vi "PROYECTO_FINAL.vi"() -> ()   [LabVIEW 2026]
uses:
  <vilib>/Instr/_visa.llb/VISA Configure Serial Port (Instr).vi
panel:
  out "MONITOR SERIAL":string
  out "ASIENTO 2 Ocupado":bool
  out "ASIENTO 1 Ocupado":bool
  out "detenido":bool
  out "volcadura":bool
  out "Velocidad GPS":dbl
  out "Humedad":dbl
  out "Temp AHT":dbl
  out "Altitud":dbl
  out "Temp BMP":dbl
  out "Presión":dbl
  out "ROLL":dbl
  out "PITCH":dbl
  out "AZ":dbl
  out "AY":dbl
  out "AX":dbl
  in  "stop":bool
  # "PROYECTO FINAL"
  # "TÓPICOS AVANZADOS \nDE SENSORES"
  # "-GARCÍA PÉREZ VÍCTOR EDUARDO\n-FRAIRE MEZA ARIATNO TOMASSI\n-NAVA ÁVILA DAVID ISAAC"
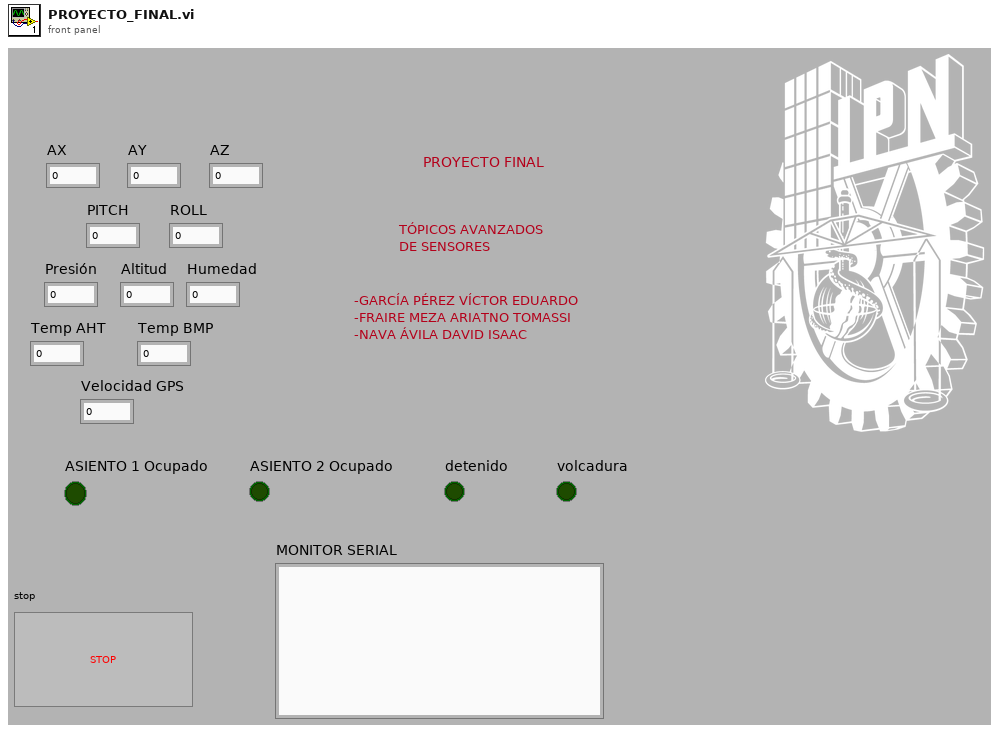
[diagram p1: front panel]
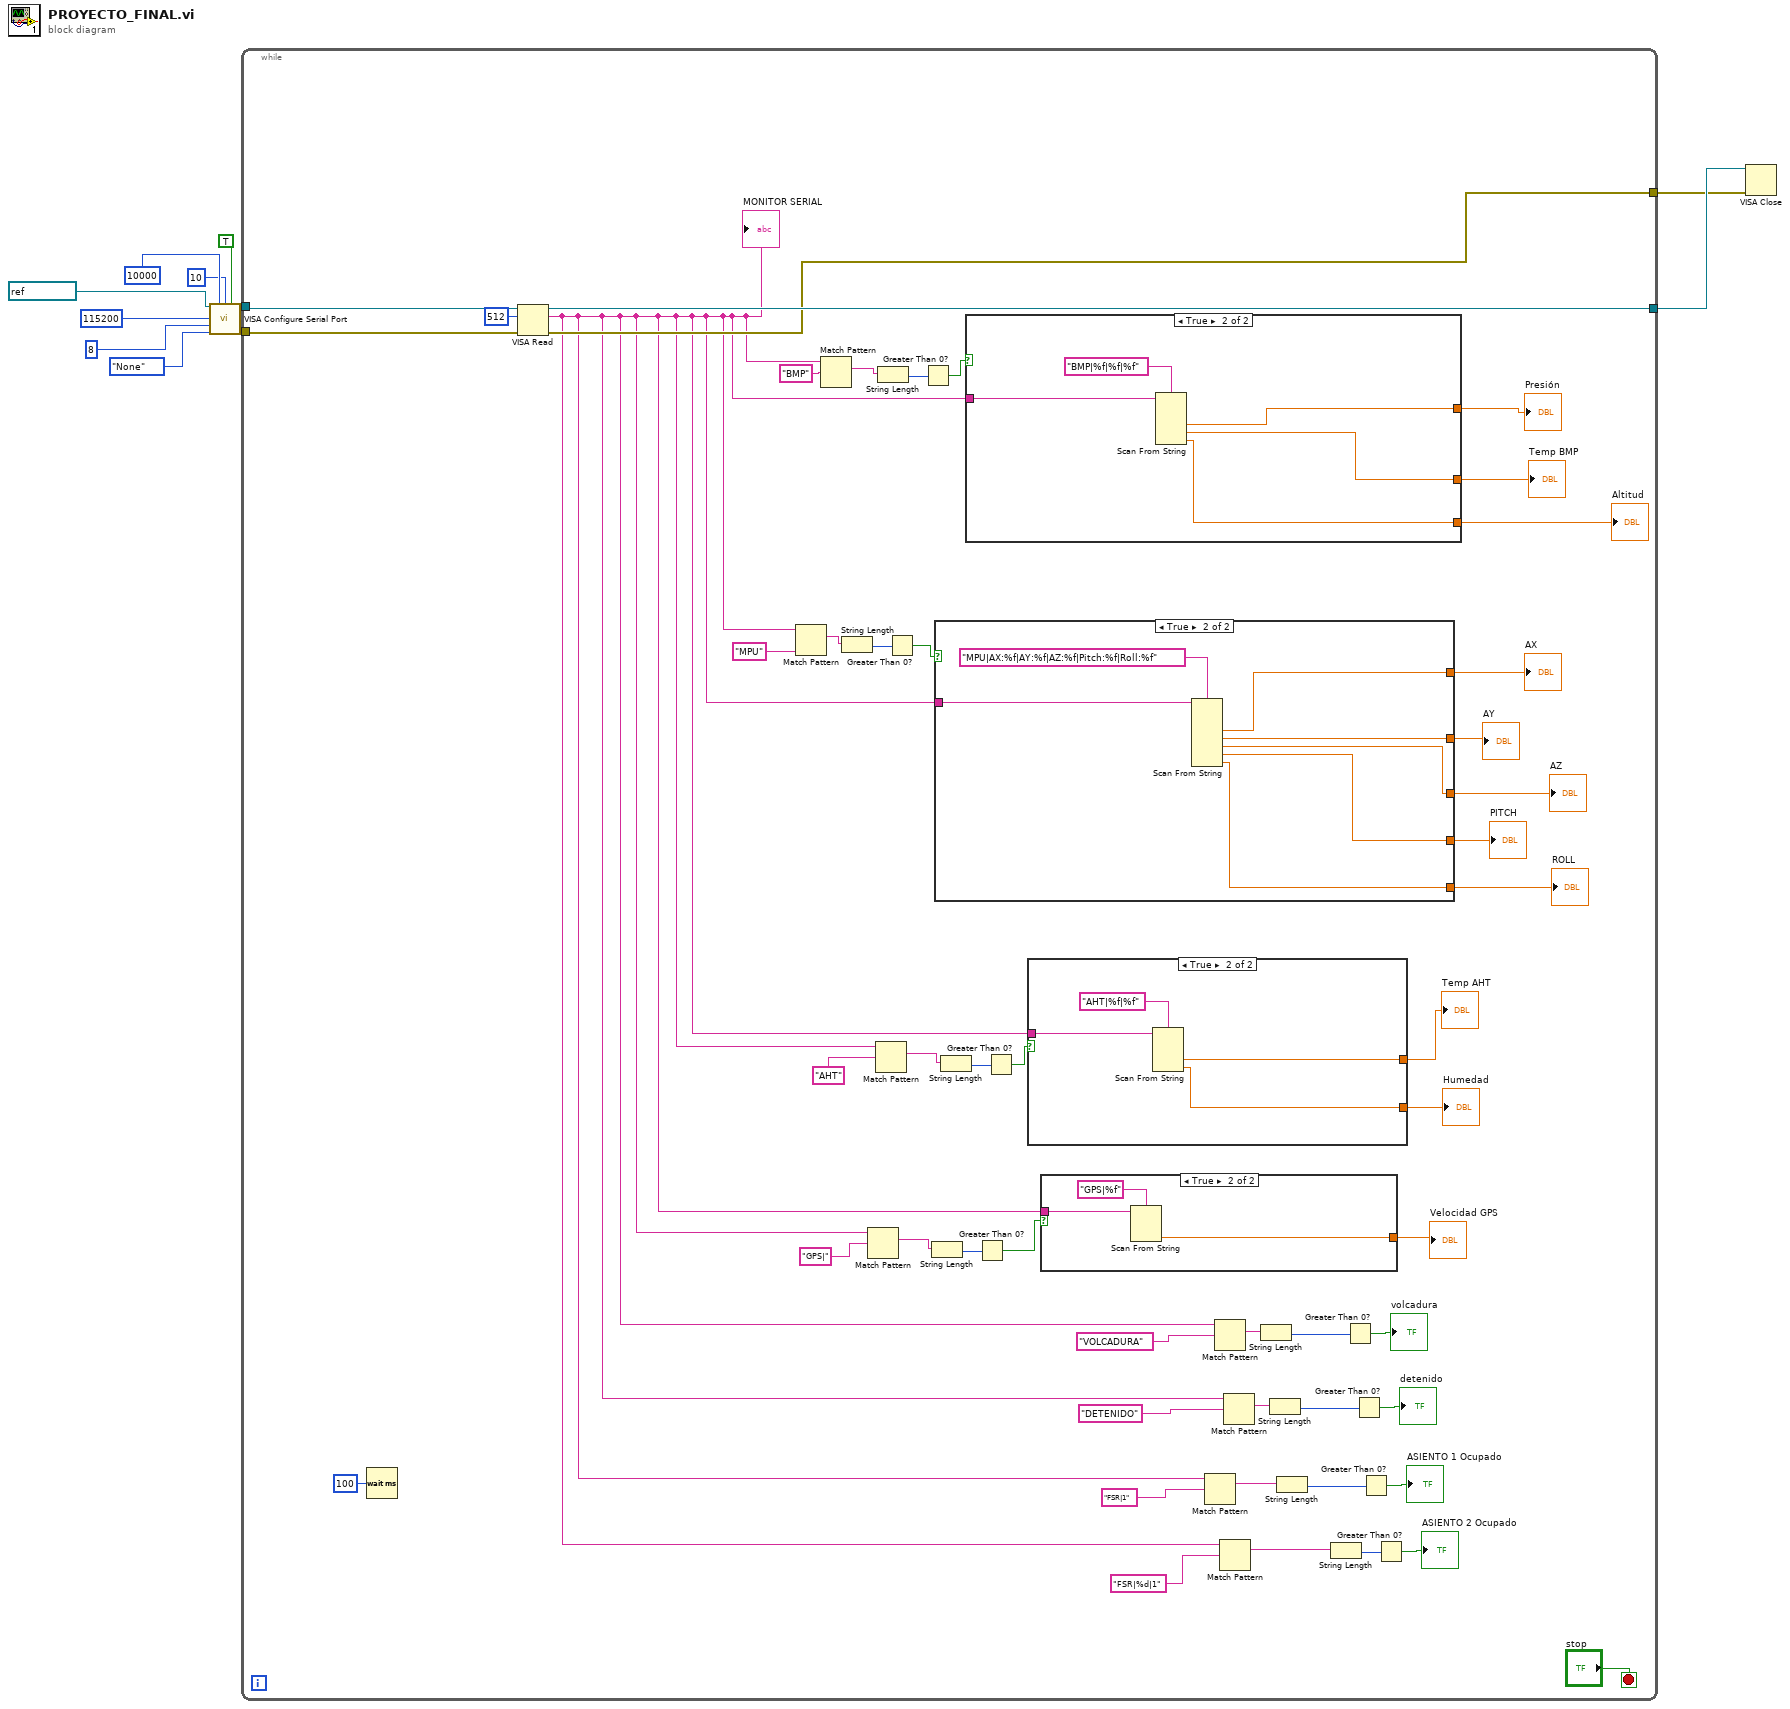
[diagram p0: block diagram]
diagram:
  n1 = call-poly "VISA Configure Serial Port"("VISA resource name"=refnum<visa-resource-name> "COM12", "timeout (10sec)"=u32 10000, "termination char\n(0xA = '\\n' = LF)"=u8 10 ("termination char\n(0xA = '\\n' = LF)"), "Enable Termination\nChar (T)"=TRUE ("Enable Termination\nChar (T)"), "baud rate (9600)"=u32 115200, "data bits (8)"=u16 8, "parity (0:none)"=enum16{"None", "Odd", "Even", "Mark", "Space"}."None") -> ("VISA resource name out"=w7:refnum<visa-resource-name>, "error out"=w6:errorcluster)  [unwired: 7 in]
  n2 = while {
    tunnel: w7 -> [w61]
    tunnel: w6 -> [w59]
    tunnel: [w27] -> w3
    tunnel: [w26] -> w2
    stop <- "stop" stop-if-true
    n3 = Wait (ms)(milliseconds to wait=u32 100) -> ()  [unwired: 1 out]
    n4 = VISA Read(VISA resource name=w61, byte count=u32 512, error in (no error)=w59) -> (VISA resource name out=w27:refnum<visa-resource-name>, read buffer=w24:string, error out=w26:errorcluster)  [unwired: 1 out]
    "MONITOR SERIAL" <- w24
    n5 = Match Pattern(string=w24, regular expression="MPU") -> (match substring=w22:string)  [unwired: 1 in, 3 out]
    n6 = Match Pattern(string=w24, regular expression="BMP") -> (match substring=w19:string)  [unwired: 1 in, 3 out]
    n7 = String Length(string=w22) -> (length=w23:i32)
    n8 = Match Pattern(string=w24, regular expression="GPS|") -> (match substring=w13:string)  [unwired: 1 in, 3 out]
    n9 = Match Pattern(string=w24, regular expression="AHT") -> (match substring=w16:string)  [unwired: 1 in, 3 out]
    n10 = String Length(string=w19) -> (length=w20:i32)
    n11 = Greater Than 0?(x=w23) -> (x > 0?=w21:bool)
    n12 = Greater Than 0?(x=w20) -> (x > 0?=w18:bool)
    n13 = String Length(string=w13) -> (length=w14:i32)
    n14 = case shown="True" w21 {
      tunnel: [_ w80] -> w38
      tunnel: [_ w79] -> w37
      tunnel: [_ w78] -> w36
      tunnel: [_ w77] -> w35
      tunnel: [_ w76] -> w34
      tunnel: w24 -> [_ w75]
      frame False {
      }
      frame True {
        n15 = Scan From String "Scan From String"(format string="MPU|AX:%f|AY:%f|AZ:%f|Pitch:%f|Roll:%f", input string=w75) -> (output 1=w80:dbl, output 2=w79:dbl, output 3=w78:dbl, output 4=w77:dbl, output 5=w76:dbl)  [unwired: 7 in, 3 out]
      }
    }
    "AX" <- w38
    "AY" <- w37
    "AZ" <- w36
    "PITCH" <- w35
    "ROLL" <- w34
    n16 = String Length(string=w16) -> (length=w17:i32)
    n17 = case shown="True" w18 {
      tunnel: [_ w73] -> w30
      tunnel: [_ w72] -> w29
      tunnel: [_ w71] -> w28
      tunnel: w24 -> [_ w70]
      frame False {
      }
      frame True {
        n18 = Scan From String(format string="BMP|%f|%f|%f", input string=w70) -> (output 1=w73:dbl, output 2=w72:dbl, output 3=w71:dbl)  [unwired: 5 in, 3 out]
      }
    }
    "Presión" <- w30
    "Temp BMP" <- w29
    "Altitud" <- w28
    n19 = Greater Than 0?(x=w14) -> (x > 0?=w12:bool)
    n20 = Greater Than 0?(x=w17) -> (x > 0?=w15:bool)
    n21 = case shown="True" w15 {
      tunnel: [_ w68] -> w33
      tunnel: [_ w67] -> w32
      tunnel: w24 -> [_ w66]
      frame False {
      }
      frame True {
        n22 = Scan From String(format string="AHT|%f|%f", input string=w66) -> (output 1=w68:dbl, output 2=w67:dbl)  [unwired: 4 in, 3 out]
      }
    }
    "Temp AHT" <- w33
    "Humedad" <- w32
    n23 = case shown="True" w12 {
      tunnel: [_ w64] -> w31
      tunnel: w24 -> [_ w63]
      frame False {
      }
      frame True {
        n24 = Scan From String(format string="GPS|%f", input string=w63) -> (output 1=w64:dbl)  [unwired: 3 in, 3 out]
      }
    }
    "Velocidad GPS" <- w31
    n25 = Match Pattern(string=w24, regular expression="FSR|1") -> (match substring=w44:string)  [unwired: 1 in, 3 out]
    n26 = Match Pattern(string=w24, regular expression="VOLCADURA") -> (match substring=w54:string)  [unwired: 1 in, 3 out]
    n27 = Match Pattern(string=w24, regular expression="FSR|%d|1") -> (match substring=w40:string)  [unwired: 1 in, 3 out]
    n28 = Match Pattern(string=w24, regular expression="DETENIDO") -> (match substring=w51:string)  [unwired: 1 in, 3 out]
    n29 = String Length(string=w54) -> (length=w52:i32)
    n30 = String Length(string=w51) -> (length=w49:i32)
    n31 = String Length(string=w44) -> (length=w45:i32)
    n32 = String Length(string=w40) -> (length=w41:i32)
    n33 = Greater Than 0?(x=w52) -> (x > 0?=→"volcadura":bool)
    n34 = Greater Than 0?(x=w49) -> (x > 0?=→"detenido":bool)
    n35 = Greater Than 0?(x=w45) -> (x > 0?=→"ASIENTO 1 Ocupado":bool)
    n36 = Greater Than 0?(x=w41) -> (x > 0?=→"ASIENTO 2 Ocupado":bool)
  }
  n37 = VISA Close(VISA resource name=w3, error in (no error)=w2) -> ()  [unwired: 1 out]
